vi "sensorNameToId.vi"(8 "error in (no error)":errorcluster, 9 "Sensor Name":string, 10 "Path":path=path "/home/ttsai/Documents/stash/ts_tcs_ofc/configData/sensorIdToName.txt", 11 "MatOper in":refnum<class "MatOper.lvclass">) -> (0 "error out":errorcluster, 2 "Sensor ID":i32, 3 "MatOper out":refnum<class "MatOper.lvclass">)   [LabVIEW 2016, in "OfcFunc.lvlib" / "MatOper.lvclass"]
doc: "Map the sensor name to ID."
uses:
  MatOper.lvclass
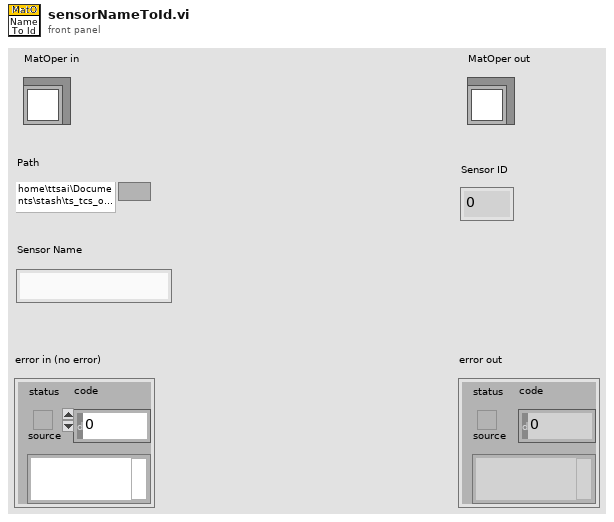
[diagram p1: front panel]
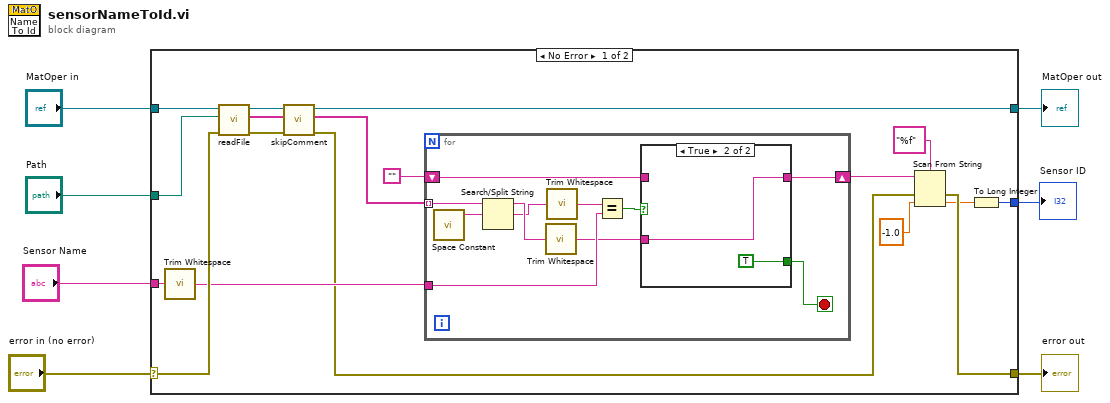
[diagram p0: block diagram]
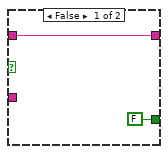
[diagram p2: hidden frame]
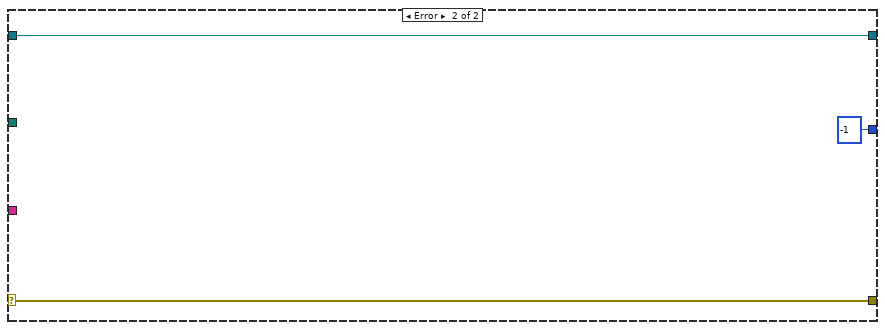
[diagram p3: hidden frame]
diagram:
  n1 = case shown="No Error" "error in (no error)" {
    selector: "error in (no error)" -> [w20 w43]
    tunnel: [w12 w43] -> w6
    tunnel: [w23 w42] -> w4
    tunnel: "MatOper in" -> [w25 w42]
    tunnel: "Path" -> [w22 _]
    tunnel: "Sensor Name" -> [w18 _]
    tunnel: [w9 -1] -> w1
    frame No Error {
      n2 = call <vilib>:"Trim Whitespace.vi"("string"=w18) -> ("trimmed string"=w15:string)  [unwired: 1 in]
      n3 = call "readFile.vi"("error in (no error)"=w20, "Path"=w22, "MatOper in"=w25) -> ("error out"=w19:errorcluster, "Array"=w21:string[], "MatOper out"=w24:refnum<class "MatOper.lvclass">)  [unwired: 6 in]
      n4 = call "skipComment.vi"("error in (no error)"=w19, "Content"=w21, "MatOper in"=w24) -> ("error out"=w13:errorcluster, "Modified Content"=w16:string[], "MatOper out"=w23:refnum<class "MatOper.lvclass">)  [unwired: 6 in]
      n5 = for {
        tunnel: w16 -> [w36] mode=indexing
        tunnel: w15 -> [w34]
        shift-right: [w30] -> w14
        shift-left: "" -> [w31]
        stop <- w32 stop-if-true
        n6 = call <vilib>:"Space Constant.vi"() -> ("String"=w35:string)
        n7 = Search/Split String(string=w36, search string/char (-)=w35) -> (substring before match=w28:string, match + rest of string=w26:string)  [unwired: 1 in, 1 out]
        n8 = call <vilib>:"Trim Whitespace.vi"("string"=w28) -> ("trimmed string"=w29:string)  [unwired: 1 in]
        n9 = call <vilib>:"Trim Whitespace.vi"("string"=w26) -> ("trimmed string"=w27:string)  [unwired: 1 in]
        n10 = Equal?(x=w27, y=w34) -> (x = y?=w33:bool)
        n11 = case shown="True" w33 {
          tunnel: [FALSE TRUE] -> w32
          tunnel: w31 -> [w37 _]
          tunnel: [w37 w39] -> w30
          tunnel: w29 -> [_ w39]
          frame False {
          }
          frame True {
          }
        }
      }
      n12 = Scan From String(format string="%f", input string=w14, error in=w13, default 1=-1.0 ("default value 1")) -> (error out=w12:errorcluster, output 1=w10:dbl)  [unwired: 1 in, 2 out]
      n13 = To Long Integer(number=w10) -> (32bit integer=w9:i32)
    }
    frame Error {
    }
  }
  "error out" <- w6
  "MatOper out" <- w4
  "Sensor ID" <- w1
